vi "Plug_in_LDA_Optimisation.vi"() -> (5 "Plug in titles":string[](array[string]), 7 "Plug in values":string[](array[string]))   [LabVIEW 2010]
uses:
  Globals/Plug_in_data_global.vi
  Globals/Meas_global.vi
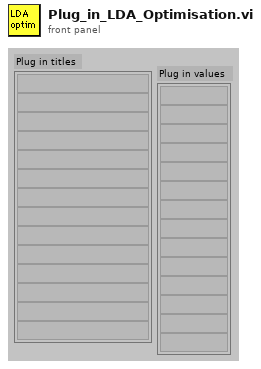
[diagram p1: front panel]
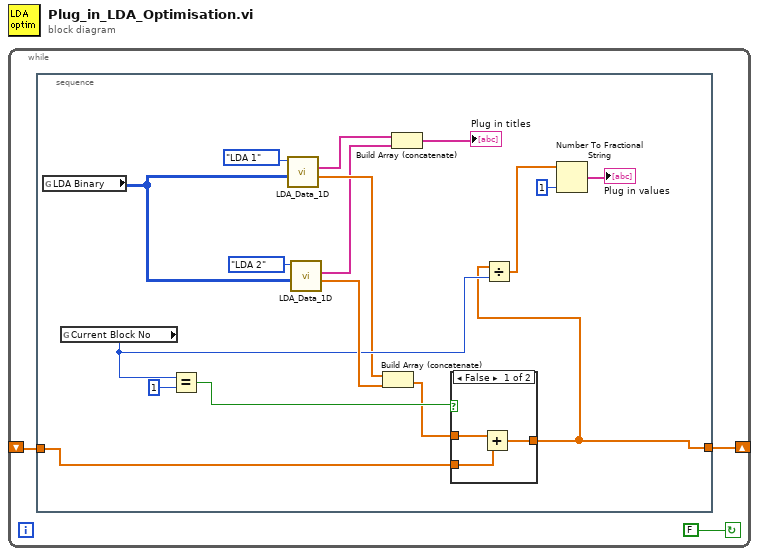
[diagram p0: block diagram]
diagram:
  n1 = while {
    shift-left: _ -> [w3]
    shift-right: [w2] -> _
    stop <- FALSE continue-if-true
    n2 = stacked-sequence {
      tunnel: w3 -> [w14]
      tunnel: [w12] -> w2
      frame #0 {
        n3 = global read "Plug_in_data_global.vi" "LDA Binary"() -> (w4:u16[][])
        n4 = global read "Meas_global.vi" "Current Block No"() -> (w13:i32)
        n5 = Equal?(x=w13, y=1) -> (x = y?=w17:bool)
        n6 = call "LDA_Data_1D.vi"("LDA Binary data"=w4, "LDA numder"=enum16{"LDA 1", "LDA 2"}."LDA 1") -> ("Results Values"=w11:dbl[], "Results titles"=w10:string[])  [unwired: 8 out]
        n7 = call "LDA_Data_1D.vi"("LDA Binary data"=w4, "LDA numder"=enum16{"LDA 1", "LDA 2"}."LDA 2") -> ("Results Values"=w16:dbl[], "Results titles"=w9:string[])  [unwired: 8 out]
        n8 = Build Array (concatenate)(w11, w16) -> (w15:dbl[])
        n9 = Build Array (concatenate)(w10, w9) -> (→"Plug in titles":string[])
        n10 = case shown="False" w17 {
          tunnel: w15 -> [w23 w24]
          tunnel: w14 -> [w22 _]
          tunnel: [w21 w24] -> w12
          frame False {
            n11 = Add(x=w23, y=w22) -> (x+y=w21:dbl[])
          }
          frame True {
          }
        }
        n12 = Divide(x=w12, y=w13) -> (x/y=w7:dbl[])
        n13 = Number To Fractional String(number=w7, precision (6)=i16 1) -> (F-format string=→"Plug in values":string[])  [unwired: 2 out]
      }
    }
  }
